vi "Auton single bo peep begin.vi"   [LabVIEW 2014]
uses:
  Robot Global Data.vi
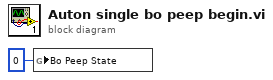
[diagram p0: block diagram]
diagram:
  n1 = global write "Robot Global Data.vi" "Bo Peep State"(i8 0 ("Bo Peep State")) -> ()
